vi "AH Bridge Initialize.vi"(6 "Read Frequency":bool, 9 "Return Dissapation":u8, 10 "Is AH2500?":bool, 11 "VISA Refnum in":refnum<visa-resource-name>) -> (1 "Frequency":dbl, 2 "Numeric":dbl, 3 "VISA Refnum out":refnum<visa-resource-name>, 4 "Wait Time (mS)":u32, 5 "Averaging Time":string[](array[string]), 7 "Setting":u32)   [LabVIEW 2019]
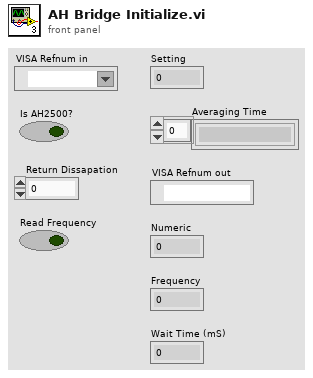
[diagram p1: front panel]
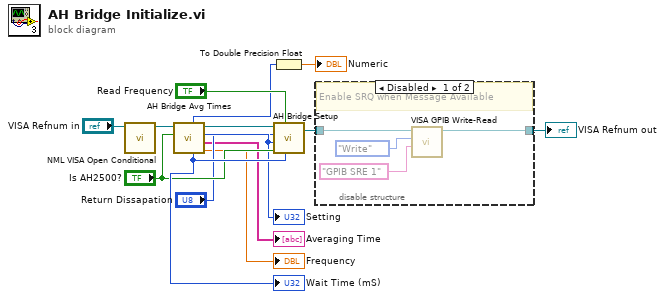
[diagram p0: block diagram]
diagram:
  n1 = call "NML VISA Open Conditional.vi"("VISA resource name"="VISA Refnum in") -> ("dup VISA Session"=w3:refnum<visa-resource-name>)  [unwired: 8 in, 2 out]
  n2 = call "AH Bridge Avg Times.vi"("VISA Resource name"=w3, "Is model 2500?"="Is AH2500?") -> ("Min Setting"=w6:u32, "Wait Time (mS)"=w14:u32, "VISA Resource out"=w10:refnum<visa-resource-name>, "Setting"=w11:u32, "Averaging Time"=→"Averaging Time":string[], "Frequency"=→"Frequency":dbl)  [unwired: 2 in]
  "Wait Time (mS)" <- w14
  "Setting" <- w11
  n3 = To Double Precision Float(number=w6) -> (double precision float=→"Numeric":dbl)
  n4 = call "AH Bridge Setup.vi"("Wait Time (mS)"=w14, "Read Frequency"="Read Frequency", "AH 2500?"="Is AH2500?", "AVE TIME"=w11, "Return Dissapation"="Return Dissapation", "Instrument Address"=w10) -> ("dup Instrument Address"=w12:refnum<visa-resource-name>)  [unwired: 1 out]
  n5 = disable-structure shown="Disabled" {
    disable-tunnel: w12 -> [w18 w19]
    disable-tunnel: [w17 w19] -> w1
    frame Disabled {
      # "Enable SRQ when Message Available"
      n6 = call "VISA GPIB Write-Read.vi"("Command"="GPIB SRE 1", "Action"=enum16{"Write", "Read", "Write & Read"}."Write", "VISA resource name"=w18) -> ("dup VISA Session"=w17:refnum<visa-resource-name>)  [unwired: 5 in, 3 out]
    }
    frame Enabled {
    }
  }
  "VISA Refnum out" <- w1
